vi "TI_INIT.vi"() -> (1 "error out":errorcluster, 2 "return":i32=666)   [LabVIEW 2011]
doc: "1. Starts the dll\n2. If successful, it leaves the VI with no error.\n3. If there is a error, the VI trys to stop and re-start the dll.\n4. If the re-start is successful, it leaves the VI with no error.\n5. If the re-start is not successful it leaves the VI with an error."
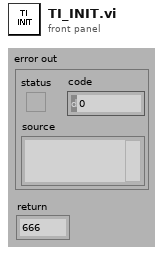
[diagram p1: front panel]
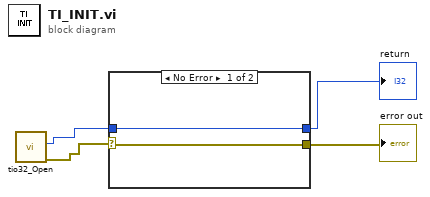
[diagram p0: block diagram]
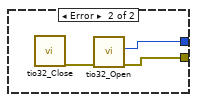
[diagram p2: hidden frame]
diagram:
  n1 = call "tio32_Open.vi"() -> ("error out"=w2:errorcluster, "return"=w1:i32)  [unwired: 6 in, 1 out]
  n2 = case shown="No Error" w2 {
    selector: w2 -> [w6 _]
    tunnel: [w6 w9] -> w4
    tunnel: [w5 w8] -> w3
    tunnel: w1 -> [w5 _]
    frame No Error {
    }
    frame Error {
      n3 = call "tio32_Close.vi"() -> ("error out"=w7:errorcluster)  [unwired: 6 in, 2 out]
      n4 = call "tio32_Open.vi"("error in (no error)"=w7) -> ("error out"=w9:errorcluster, "return"=w8:i32)  [unwired: 5 in, 1 out]
    }
  }
  "error out" <- w4
  "return" <- w3
